vi "Found to Used instruments.vi"(8 "error in (no error)":errorcluster, 11 "Test Framework in":refnum<class "Test Framework.lvclass">) -> (0 "error out":errorcluster, 3 "Test Framework out":refnum<class "Test Framework.lvclass">)   [LabVIEW 2020, in "Test Framework.lvclass"]
uses:
  Test Framework.lvclass
  Instruments/Power Supply/Power Supply.lvclass
  C:/Sandbox/RF Bench/Source Code/WiSpry Test Framework/Instruments/Instrument.lvclass
  Instruments/Power Meter/Power Meter.lvclass
  Instruments/Instrument.lvclass
  Instruments/Path Switch/Path Switch.lvclass
  Instruments/Controls/Interface String Cluster.ctl
  Instruments/Instrument.lvclass/Instrument.ctl
  Instruments/Power Supply/Power Supply.lvclass/Power Supply.ctl
  Test Framework.lvclass/Test Framework.ctl
  <vilib>/Utility/config.llb/Read Key (String).vi
  <vilib>/Utility/config.llb/Read Key (I32).vi
  Devices/Device.lvclass
  <vilib>/Utility/config.llb/NI_LVConfig.lvlib
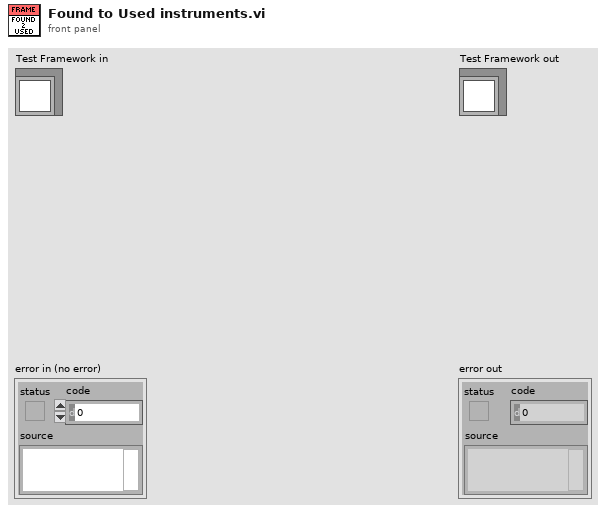
[diagram p1: front panel]
types:
  T1 = cluster{"Instrument Name":string, "Instrument.lvclass":refnum<class "Instrument.lvclass">, "Reference":bool}[]
  T2 = cluster{"Instrument Name":string, "Instrument.lvclass":refnum<class "Instrument.lvclass">, "Reference":bool}
  T3 = typedef "Instrument.lvclass/Interface String Cluster.ctl" = cluster{"Interface":string, "IDN string":string, "Instance":i32}
  T4 = typedef "Test Framework.lvclass/Reference Selector.ctl" = enum16{"Signal Generator 1", "Signal Generator 2", "Spectrum Analyzer"}
  T5 = cluster{"Found Instruments":string[][], "Reference Selected":T4}
  T6 = typedef "NI_LVConfig.lvlib/Config Data RefNum.ctl" = refnum<k1>
  T7 = cluster{string, "Instrument out":refnum<class "Instrument.lvclass">, bool}
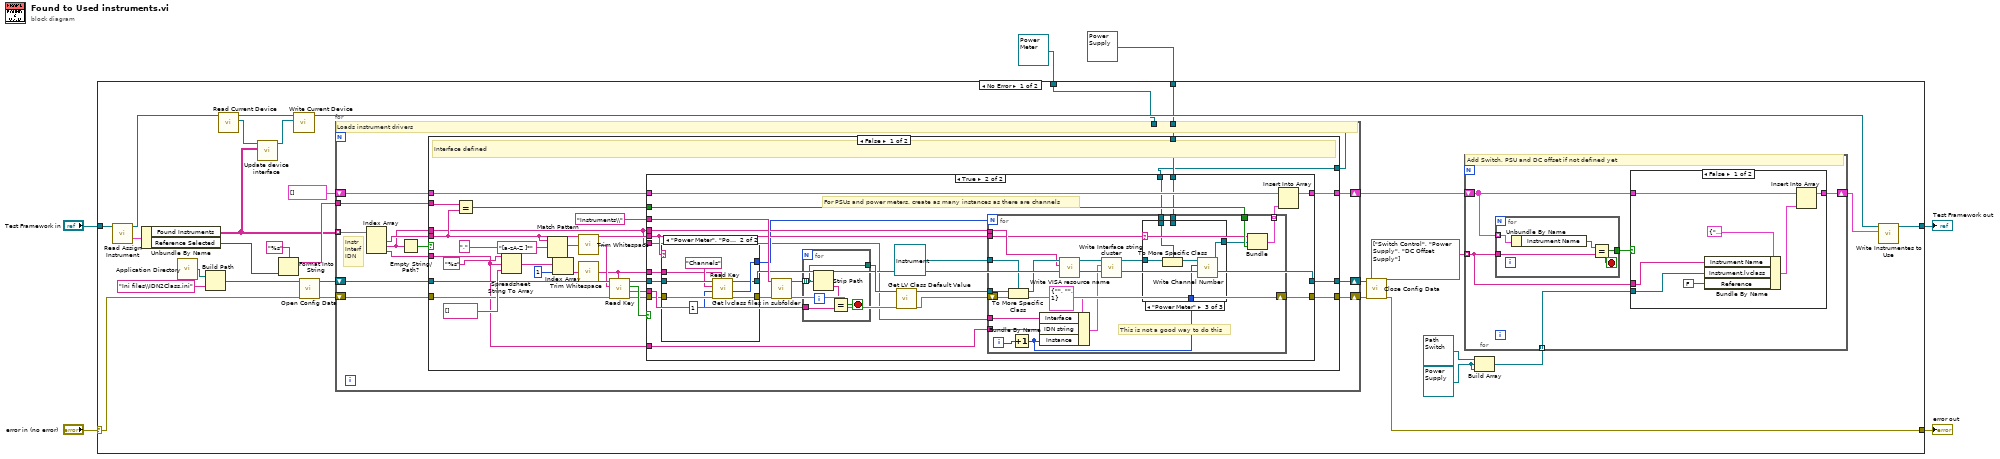
[diagram p0: block diagram]
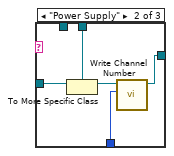
[diagram p5: hidden frame]
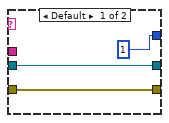
[diagram p6: hidden frame]
diagram:
  n1 = case shown="No Error" "error in (no error)" {
    selector: "error in (no error)" -> [w30 w174]
    tunnel: [w12 w174] -> w5
    tunnel: [w28 w173] -> w3
    tunnel: "Test Framework in" -> [w36 w173]
    tunnel: refnum<class "Power Supply.lvclass"> refnum ("Power Supply.lvclass") -> [w11 _]
    tunnel: refnum<class "Power Meter.lvclass"> refnum ("Power Meter.lvclass") -> [w8 _]
    frame No Error {
      w15 = refnum<class "Power Supply.lvclass"> refnum ("Power Supply.lvclass")
      n2 = call-dynamic "Read Assign Instrument.vi"("Test Framework in"=w36) -> ("Assign Instrument"=w35:T5, "Test Framework out"=w21:refnum<class "Test Framework.lvclass">)  [unwired: 9 in]
      n3 = Unbundle By Name(w35) -> ("Found Instruments"=w7:string[][], "Reference Selected"=w18:T4)
      n4 = call <vilib>:"Application Directory.vi"() -> ("Application Directory"=w34:path)
      n5 = Build Path(base path=w34, name or relative path="Ini files\\IDN2Class.ini") -> (appended path=w32:path)
      n6 = call-dynamic "Read Current Device.vi"("Test Framework in"=w21) -> ("Current Device.lvclass"=w10:refnum<class "Device.lvclass">, "Test Framework out"=w20:refnum<class "Test Framework.lvclass">)  [unwired: 9 in]
      n7 = call-dynamic "Update device interface.vi"("Found Instruments"=w7, "Device in"=w10) -> ("Device out"=w9:refnum<class "Device.lvclass">)  [unwired: 8 in, 1 out]
      n8 = Format Into String(format string="%s", w18) -> (resulting string=w16:string)  [unwired: 2 in, 1 out]
      n9 = call-dynamic "Write Current Device.vi"("Current Device.lvclass"=w9, "Test Framework in"=w20) -> ("Test Framework out"=w19:refnum<class "Test Framework.lvclass">)  [unwired: 9 in]
      n10 = call <vilib>:"Open Config Data.vi"("error in (no error)"=w30, "configuration file path"=w32) -> ("error out"=w31:errorcluster, "refnum"=w27:T6)  [unwired: 7 in, 1 out]
      n11 = for {
        tunnel: w7 -> [w67] mode=indexing
        shift-right: [w61] -> w13
        shift-left: w31 -> [w62]
        shift-right: [w58] -> w26
        shift-left: T1 [] ("Instrumentes to Use") -> [w59]
        tunnel: w16 -> [w57]
        shift-right: [w56] -> w14
        shift-left: w27 -> [w63]
        tunnel: w11 -> [w55]
        tunnel: w8 -> [w54]
        # "Instr\nInterf\nIDN"
        # "Loads instrument drivers"
        n12 = Index Array(array=w67) -> (element #1=w65:string, element #2=w60:string, element #3=w64:string)  [unwired: 3 in]
        n13 = Empty String/Path?(string/path=w60) -> (empty?=w66:bool)
        n14 = case shown="False" w66 {
          tunnel: w65 -> [w77 _]
          tunnel: w64 -> [w71 _]
          tunnel: w63 -> [w91 w170]
          tunnel: w62 -> [w92 w172]
          tunnel: [w85 w172] -> w61
          tunnel: w60 -> [w72 _]
          tunnel: w59 -> [w87 w171]
          tunnel: [w86 w171] -> w58
          tunnel: w57 -> [w78 _]
          tunnel: [w73 w170] -> w56
          tunnel: w55 -> [w69 _]
          tunnel: w54 -> [w68 _]
          frame False {
            # "Interface defined"
            n15 = Equal?(x=w78, y=w77) -> (x = y?=w76:bool)
            n16 = Spreadsheet String To Array(delimiter (Tab)=",", format string="%s" ("spreadsheet string"), spreadsheet string=w71, array type (2D Dbl)=string[] []) -> (array=w93:string[])
            n17 = Match Pattern(string=w77, regular expression="[a-zA-Z ]*") -> (match substring=w82:string)  [unwired: 1 in, 3 out]
            n18 = Index Array(array=w93, index=1) -> (element=w80:string)
            n19 = call <vilib>:"Trim Whitespace.vi"("string"=w80) -> ("trimmed string"=w70:string)  [unwired: 1 in]
            n20 = call <vilib>:"Trim Whitespace.vi"("string"=w82) -> ("trimmed string"=w79:string)  [unwired: 1 in]
            n21 = call-poly <vilib>:"Read Key.vi"("section"=w70, "error in (no error)"=w92, "key"=w79, "refnum"=w91) -> ("error out"=w89:errorcluster, "value"=w88:string, "found?"=w90:bool, "refnum out"=w74:T6)  [unwired: 4 in]
            n22 = case shown="True" w90 {
              tunnel: w89 -> [w97 w107]
              tunnel: w88 -> [_ w121]
              tunnel: "Instruments\\" ("string") -> [_ w123]
              tunnel: w72 -> [_ w110]
              tunnel: w77 -> [_ w109]
              tunnel: w87 -> [w98 w115]
              tunnel: [w98 w114] -> w86
              tunnel: [w97 w112] -> w85
              tunnel: w76 -> [_ w111]
              tunnel: w71 -> [_ w102]
              tunnel: w74 -> [w96 w108]
              tunnel: [w96 w105] -> w73
              tunnel: w72 -> [_ w103]
              tunnel: w70 -> [_ w101]
              tunnel: w69 -> [_ w100]
              tunnel: w68 -> [_ w99]
              frame False {
              }
              frame True {
                # "For PSUs and power meters, create as many instances as there are channels"
                n23 = case shown="\"Power Meter\", \"Power Supply\"" w109 {
                  tunnel: w108 -> [w155 w165]
                  tunnel: w107 -> [w157 w164]
                  tunnel: [w157 w163] -> w106
                  tunnel: [1 w162] -> w104
                  tunnel: [w155 w160] -> w105
                  tunnel: w101 -> [_ w158]
                  frame Default {
                  }
                  frame "Power Meter", "Power Supply" {
                    n24 = call-poly <vilib>:"Read Key.vi"("section"=w158, "error in (no error)"=w164, "default value"=1, "key"="Channels", "refnum"=w165) -> ("error out"=w163:errorcluster, "value"=w162:i32, "refnum out"=w160:T6)  [unwired: 3 in, 1 out]
                  }
                }
                n25 = call "Get lvclass files in subfolder.vi"("Error In"=w106, "Sub Folder"=w123) -> ("Error Out"=w120:errorcluster, "Found lvclass files"=w122:path[])  [unwired: 8 in]
                n26 = for {
                  tunnel: w122 -> [w166] mode=indexing
                  tunnel: w121 -> [w168]
                  tunnel: [w166] -> w119
                  stop <- w167 stop-if-true
                  n27 = Strip Path(path=w166) -> (name=w169:string)  [unwired: 1 out]
                  n28 = Equal?(x=w169, y=w168) -> (x = y?=w167:bool)
                }
                n29 = call <vilib>:"Get LV Class Default Value.vi"("error in (no error)"=w120, "class path"=w119) -> ("error out"=w118:errorcluster, "object"=w117:refnum<class>)  [unwired: 8 in]
                n30 = for {
                  N: w104 -> [_]
                  tunnel: w117 -> [w142]
                  tunnel: refnum<class "Instrument.lvclass"> refnum ("Instrument.lvclass") -> [w141]
                  tunnel: [w139] -> w113 mode=indexing
                  tunnel: w111 -> [w137]
                  tunnel: w110 -> [w135]
                  tunnel: w109 -> [w129]
                  shift-right: [w138] -> w112
                  shift-left: w118 -> [w143]
                  tunnel: w103 -> [w134]
                  tunnel: w102 -> [w133]
                  tunnel: w100 -> [w126]
                  tunnel: w99 -> [w124]
                  i -> [w131]
                  # "This is not a good way to do this"
                  n31 = To More Specific Class(target class=w141, reference=w142, error in=w143) -> (specific class reference=w140:refnum<class "Instrument.lvclass">, error out=w138:errorcluster)
                  n32 = Increment(x=w131) -> (x+1=w125:i32)
                  n33 = Bundle By Name(cluster=T3 {"Interface"="", "IDN string"="", "Instance"=1} ("Interface sting cluster"), "Interface"=w134, "IDN string"=w133, "Instance"=w125) -> (w132:T3)
                  n34 = call "Write VISA resource name.vi"("VISA resource name"=w135, "Instrument in"=w140) -> ("Instrument out"=w136:refnum<class "Instrument.lvclass">)  [unwired: 9 in]
                  n35 = call "Write Interface string cluster.vi"("Interface sting cluster"=w132, "Instrument in"=w136) -> ("Instrument out"=w128:refnum<class "Instrument.lvclass">)  [unwired: 9 in]
                  n36 = case shown="\"Power Meter\"" w129 {
                    tunnel: w128 -> [w144 w148 w154]
                    tunnel: [w144 w149 w151] -> w127
                    tunnel: w126 -> [_ w146 _]
                    tunnel: w125 -> [_ w145 w150]
                    tunnel: w124 -> [_ _ w153]
                    frame Default {
                    }
                    frame "Power Supply" {
                      n37 = To More Specific Class(target class=w146, reference=w148) -> (specific class reference=w147:refnum<class "Power Supply.lvclass">)  [unwired: 1 in, 1 out]
                      n38 = call "Write Channel Number.vi"("Channel Number"=w145, "Power Supply in"=w147) -> ("Power Supply out"=w149:refnum<class "Power Supply.lvclass">)  [unwired: 9 in]
                    }
                    frame "Power Meter" {
                      n39 = To More Specific Class(target class=w153, reference=w154) -> (specific class reference=w152:refnum<class "Power Meter.lvclass">)  [unwired: 1 in, 1 out]
                      n40 = call-dynamic "Write Channel Number.vi"("Channel Number"=w150, "Power Meter in"=w152) -> ("Power Meter out"=w151:refnum<class "Power Meter.lvclass">)  [unwired: 9 in]
                    }
                  }
                  n41 = Bundle(w129, "Instrument out"=w127, w137) -> (w139:T7)  [unwired: 1 in]
                }
                n42 = Insert Into Array(array=w115, new element=w113) -> (w114:T1)  [unwired: 1 in]
              }
            }
          }
          frame True {
            # "No Interface defined ignore"
          }
        }
      }
      n43 = call <vilib>:"Close Config Data.vi"("error in (no error)"=w13, "refnum"=w14) -> ("error out"=w12:errorcluster)  [unwired: 8 in, 1 out]
      n44 = Build Array(refnum<class "Path Switch.lvclass"> refnum ("Path Switch.lvclass"), w15, w15) -> (w22:refnum<class "Instrument.lvclass">[])
      n45 = for {
        shift-right: [w39] -> w25
        shift-left: w26 -> [w40]
        tunnel: string[] ["Switch Control", "Power Supply", "DC Offset Supply"] -> [w38] mode=indexing
        tunnel: w22 -> [w37] mode=indexing
        # "Add Switch, PSU and DC offset if not defined yet"
        n46 = for {
          tunnel: w40 -> [w53] mode=indexing
          tunnel: [w51] -> w41
          tunnel: w38 -> [w50]
          stop <- w51 stop-if-true
          n47 = Unbundle By Name(w53) -> ("Instrument Name"=w52:string)
          n48 = Equal?(x=w52, y=w50) -> (x = y?=w51:bool)
        }
        n49 = case shown="False" w41 {
          tunnel: w40 -> [w48 w49]
          tunnel: [w47 w49] -> w39
          tunnel: w38 -> [w46 _]
          tunnel: w37 -> [w45 _]
          frame False {
            n50 = Bundle By Name(cluster=T2 {"Instrument Name"="", "Instrument.lvclass"=refnum, "Reference"=FALSE} ("new element/subarray"), "Instrument Name"=w46, "Instrument.lvclass"=w45, "Reference"=FALSE) -> (w43:T2)
            n51 = Insert Into Array(array=w48, new element=w43) -> (w47:T1)  [unwired: 1 in]
          }
          frame True {
          }
        }
      }
      n52 = call "Write Instrumentes to Use.vi"("Instruments to Use"=w25, "Test Framework in"=w19) -> ("Test Framework out"=w28:refnum<class "Test Framework.lvclass">)  [unwired: 9 in]
    }
    frame Error {
    }
  }
  "error out" <- w5
  "Test Framework out" <- w3
